vi "ReadPin.vi"(8 "error in (no error)":errorcluster, 9 "Pin":dbl, 10 "Port":dbl, 11 "Simulado in":refnum<class "Simulado.lvclass">) -> (0 "error out":errorcluster, 3 "Simulado out":refnum<class "Simulado.lvclass">)   [LabVIEW 2020, in "Simulado.lvclass"]
uses:
  Simulado.lvclass
  Simulado.lvclass/Simulado.ctl
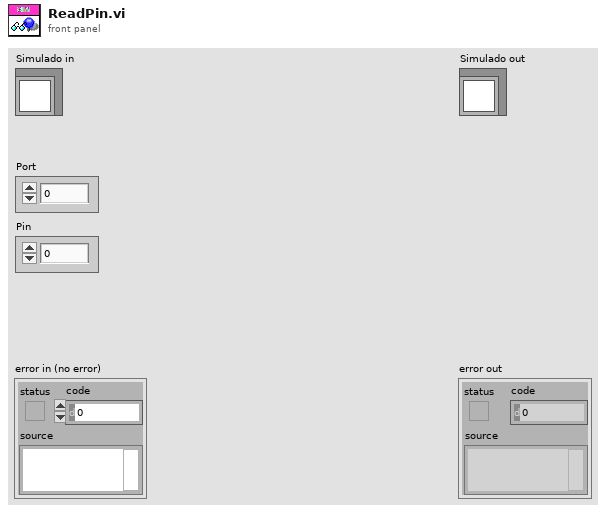
[diagram p1: front panel]
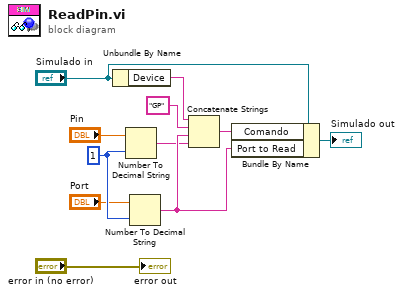
[diagram p0: block diagram]
diagram:
  w7 = i16 1 ("width (-)")
  n1 = Unbundle By Name("Simulado in") -> ("Device"=w10:string)
  n2 = Number To Decimal String(number="Pin", width (-)=w7) -> (decimal integer string=w6:string)
  n3 = Number To Decimal String(number="Port", width (-)=w7) -> (decimal integer string=w8:string)
  n4 = Concatenate Strings(w10, "GP" ("string"), w8, w6) -> (w9:string)
  n5 = Bundle By Name(cluster="Simulado in", "Comando"=w9, "Port to Read"=w8) -> (→"Simulado out":refnum<class "Simulado.lvclass">)
  "error out" <- "error in (no error)"
